vi "Programa de labview.vi"() -> ()   [LabVIEW 2012]
uses:
  <vilib>/Instr/_visa.llb/Select Event Type.ctl
panel:
  in  "VISA resource name":refnum<visa-resource-name>
  in  "stop":bool
  out "Byte recibido":u16
  out "Byte enviado":u32
  out "Datos recibidos":u8[](array[numeric])
  in  "LED":bool
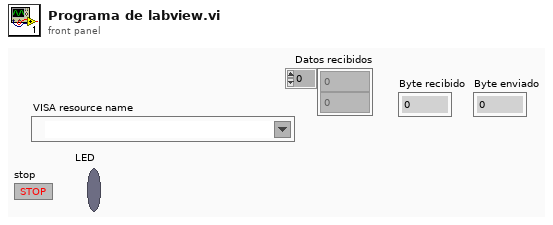
[diagram p1: front panel]
types:
  T1 = typedef "Select Event Type.ctl" = u32
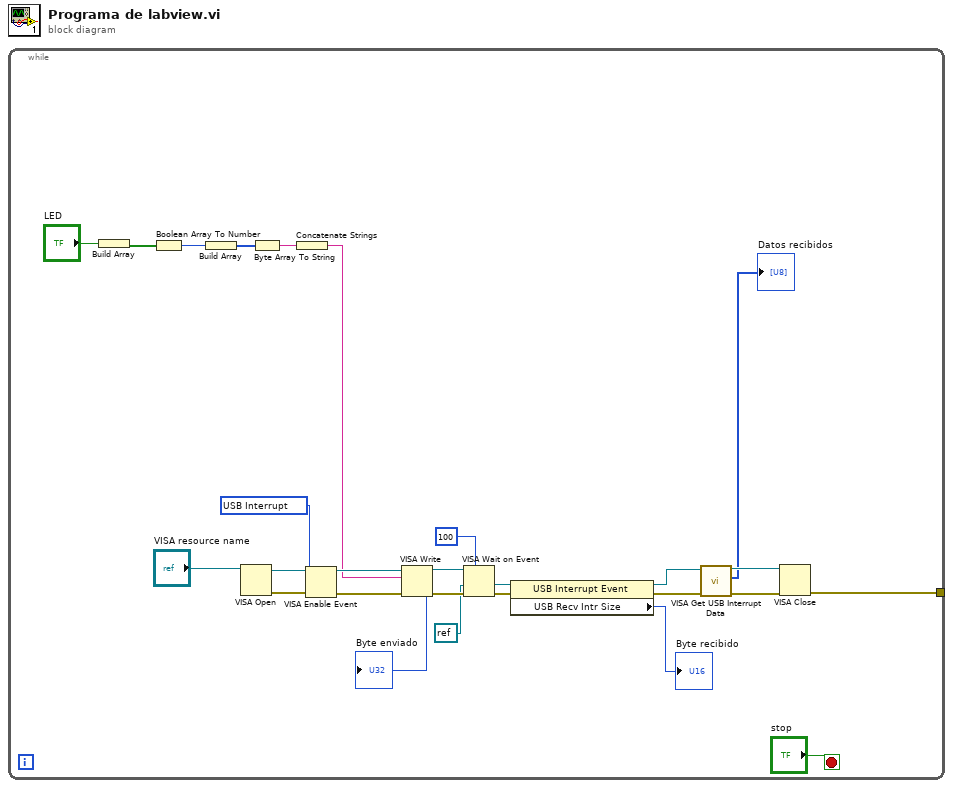
[diagram p0: block diagram]
diagram:
  n1 = while {
    tunnel: [w13] -> _
    stop <- "stop" stop-if-true
    w7 = T1 1073684535 items=["Service Request"=1073684491, "Trigger"=3221168138, "Clear"=1073684493, "VXI Signal"=1073684512, "VXI/VME Interrupt"=3221168161, "VXI/VME Sysfail"=1073684509, "VXI/VME Sysreset"=1073684510, "GPIB CIC"=1073684498, "GPIB Talk"=1073684499, "GPIB Listen"=1073684500, "PXI Interrupt"=1073684514, "Serial Break"=1073684515, "Serial TermChar"=1073684516, "Serial CTS"=1073684521, "Serial DSR"=1073684522, "Serial DCD"=1073684524, "Serial RI"=1073684526, "Serial Character"=1073684533, "USB Interrupt"=1073684535, "All Enabled"=1073709055] ("Event Type")
    n2 = Build Array("LED") -> (w19:bool[])
    n3 = Boolean Array To Number(Boolean array=w19) -> (number=w17:u32)
    n4 = Build Array(w17) -> (w18:u32[])
    n5 = VISA Open(VISA resource name="VISA resource name") -> (VISA resource name=w11:refnum<visa-resource-name>, error out=w10:errorcluster)  [unwired: 4 in]
    n6 = Byte Array To String(unsigned byte array=w18) -> (string=w5:string)
    n7 = Concatenate Strings(w5) -> (w2:string)
    n8 = VISA Enable Event(8:w10, 10:w7, 11:w11) -> (0:w8:errorcluster, 3:w9:refnum<visa-resource-name>)  [unwired: 1 in]
    n9 = VISA Write(VISA resource name=w9, write buffer=w2, error in (no error)=w8) -> (VISA resource name out=w26:refnum<visa-resource-name>, return count=→"Byte enviado":u32, error out=w12:errorcluster)
    n10 = VISA Wait on Event(7:u32 100 ("General Settings:Timeout Value"), 8:w12, 9:refnum<visa-resource-name> refnum ("event class (Generic Event)"), 11:w26) -> (0:w25:errorcluster, 1:w4:refnum<visa-resource-name>)  [unwired: 1 in, 2 out]
    n11 = property class="USB Interrupt Event"(reference=w4, error in=w25) -> (reference out=w21:refnum<visa-resource-name>, error out=w22:errorcluster, "USB Recv Intr Size"=→"Byte recibido":u16)
    n12 = call <vilib>:"VISA Get USB Interrupt Data.vi"("error in (no error)"=w22, "VISA USB Intr Event"=w21) -> ("error out"=w14:errorcluster, "data buffer"=→"Datos recibidos":u8[], "VISA USB Intr Event out"=w15:refnum<visa-resource-name>)  [unwired: 7 in]
    n13 = VISA Close(VISA resource name=w15, error in (no error)=w14) -> (error out=w13:errorcluster)
  }
